vi "Setup.vi"(11 "Application in":refnum<class "Application.lvclass">) -> (0 "error out":errorcluster, 3 "Application out":refnum<class "Application.lvclass">)   [LabVIEW 2017, in "Application.lvclass"]
doc: "Application.lvclass:Setup.vi does nothing. Child classes should override this VI with any work needed to setup the main body of the execution. This includes requesting resources that will be needed for the entire duration of the execution and reading any configuration files. Child classes are not required to do anything during Setup as there are plenty of apps that can jump straight into their main execution logic."
uses:
  Application.lvclass
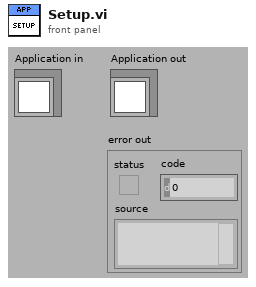
[diagram p1: front panel]
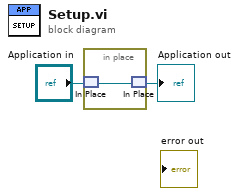
[diagram p0: block diagram]
diagram:
  n1 = in-place {
    n2 = in-place-match #1("Application in") -> (w3:refnum<class "Application.lvclass">)
    n3 = in-place-match #1(w3) -> (→"Application out":refnum<class "Application.lvclass">)
  }
